vi "Read.vi"(8 "error in (no error)":errorcluster, 11 "Start Log Command Config in":refnum<class "Start Log Command Config.lvclass">) -> (0 "error out":errorcluster, 2 "Test":string, 3 "Start Log Command Config out":refnum<class "Start Log Command Config.lvclass">)   [LabVIEW 2020, in "VolatusSeqConfig.lvlib" / "Start Log Command Config.lvclass"]
uses:
  Start Log Command Config.lvclass
  Start Log Command Config.lvclass/Start Log Command Config.ctl
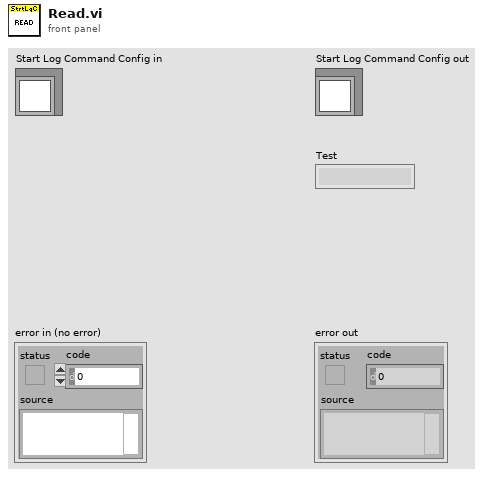
[diagram p1: front panel]
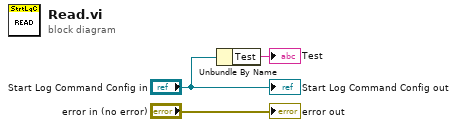
[diagram p0: block diagram]
diagram:
  n1 = Unbundle By Name("Start Log Command Config in") -> ("Test"=→"Test":string)
  "error out" <- "error in (no error)"
  "Start Log Command Config out" <- "Start Log Command Config in"
